vi "Reset Gas Meter.vi"(7 "Ritter Gas Drum Meter":bool, 8 "error in (no error)":errorcluster, 10 "Ritter Gas Meter 1":refnum<visa-resource-name>, 11 "Gas Meter 1":refnum<visa-resource-name>) -> (0 "error out":errorcluster)   [LabVIEW 2023]
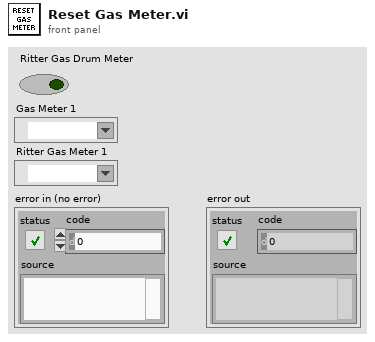
[diagram p1: front panel]
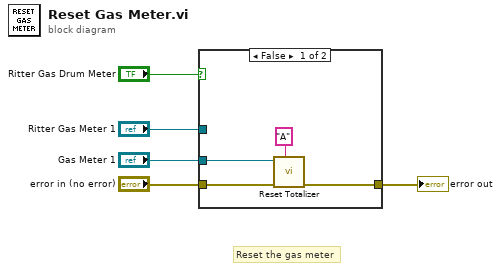
[diagram p0: block diagram]
diagram:
  # "Reset the gas meter"
  n1 = case shown="False" "Ritter Gas Drum Meter" {
    tunnel: "error in (no error)" -> [w9 _]
    tunnel: [w8 _] -> w3
    tunnel: "Gas Meter 1" -> [w7 _]
    tunnel: "Ritter Gas Meter 1" -> [_ _]
    frame False {
      n2 = call "Reset Totalizer.vi"("Unit ID (A)"="A", "error in"=w9, "VISA Session In"=w7) -> ("error out"=w8:errorcluster)  [unwired: 6 in, 2 out]
    }
    frame True {
    }
  }
  "error out" <- w3
